vi "loggin'_begin.vi"   [LabVIEW 2018]
uses:
  <userlib>/836-Library/System/QCP_V2/QCPSupportCode/QCPData.ctl
types:
  T1 = typedef "QCP_RefNum.ctl" = cluster{"Data Value Refnum":refnum<data-value>, "semaphore":T2}
  T2 = typedef "Semaphore RefNum" = refnum<k1>
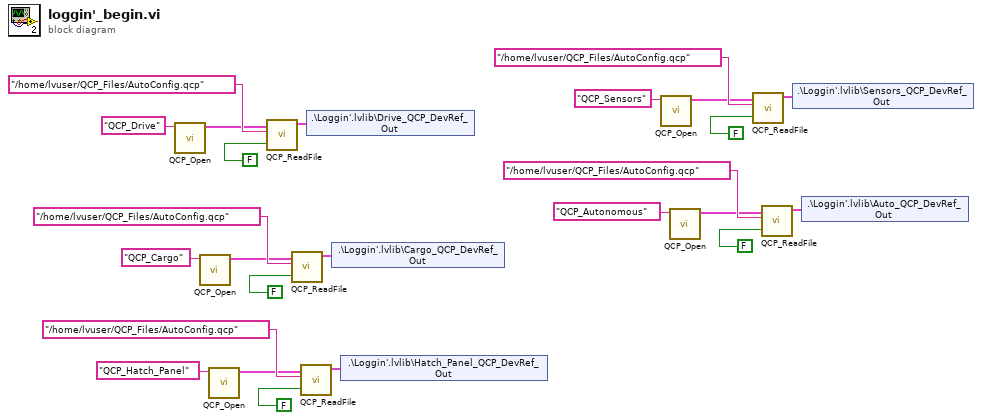
[diagram p0: block diagram]
diagram:
  n1 = call <userlib>:"QCP_Open.vi"("Name"="QCP_Drive") -> ("QCP_DevRef_Out"=w23:T1)  [unwired: 9 in, 1 out]
  n2 = call <userlib>:"QCP_Open.vi"("Name"="QCP_Cargo") -> ("QCP_DevRef_Out"=w19:T1)  [unwired: 9 in, 1 out]
  n3 = call <userlib>:"QCP_Open.vi"("Name"="QCP_Hatch_Panel") -> ("QCP_DevRef_Out"=w15:T1)  [unwired: 9 in, 1 out]
  n4 = call <userlib>:"QCP_ReadFile.vi"("Overrite Existing Data?"=FALSE, "Path"="/home/lvuser/QCP_Files/AutoConfig.qcp", "QCP_DevRef_In"=w23) -> ("QCP_DevRef_Out"=w5:T1)  [unwired: 7 in, 1 out]
  n5 = call <userlib>:"QCP_ReadFile.vi"("Overrite Existing Data?"=FALSE, "Path"="/home/lvuser/QCP_Files/AutoConfig.qcp", "QCP_DevRef_In"=w19) -> ("QCP_DevRef_Out"=w4:T1)  [unwired: 7 in, 1 out]
  n6 = call <userlib>:"QCP_ReadFile.vi"("Overrite Existing Data?"=FALSE, "Path"="/home/lvuser/QCP_Files/AutoConfig.qcp", "QCP_DevRef_In"=w15) -> ("QCP_DevRef_Out"=w3:T1)  [unwired: 7 in, 1 out]
  n7 = shared-variable ".\\Loggin'.lvlib\\Drive_QCP_DevRef_Out"(w5) -> ()  [unwired: 1 in, 1 out]
  n8 = shared-variable ".\\Loggin'.lvlib\\Cargo_QCP_DevRef_Out"(w4) -> ()  [unwired: 1 in, 1 out]
  n9 = shared-variable ".\\Loggin'.lvlib\\Hatch_Panel_QCP_DevRef_Out"(w3) -> ()  [unwired: 1 in, 1 out]
  n10 = call <userlib>:"QCP_Open.vi"("Name"="QCP_Sensors") -> ("QCP_DevRef_Out"=w11:T1)  [unwired: 9 in, 1 out]
  n11 = call <userlib>:"QCP_Open.vi"("Name"="QCP_Autonomous") -> ("QCP_DevRef_Out"=w7:T1)  [unwired: 9 in, 1 out]
  n12 = call <userlib>:"QCP_ReadFile.vi"("Overrite Existing Data?"=FALSE, "Path"="/home/lvuser/QCP_Files/AutoConfig.qcp", "QCP_DevRef_In"=w11) -> ("QCP_DevRef_Out"=w2:T1)  [unwired: 7 in, 1 out]
  n13 = call <userlib>:"QCP_ReadFile.vi"("Overrite Existing Data?"=FALSE, "Path"="/home/lvuser/QCP_Files/AutoConfig.qcp", "QCP_DevRef_In"=w7) -> ("QCP_DevRef_Out"=w1:T1)  [unwired: 7 in, 1 out]
  n14 = shared-variable ".\\Loggin'.lvlib\\Sensors_QCP_DevRef_Out"(w2) -> ()  [unwired: 1 in, 1 out]
  n15 = shared-variable ".\\Loggin'.lvlib\\Auto_QCP_DevRef_Out"(w1) -> ()  [unwired: 1 in, 1 out]
